vi "Write Registers to write.vi"(10 "Registers to write":T1[](array[typedef]), 11 "Device in":refnum<class "PIC-Device.lvclass">) -> (3 "Device out":refnum<class "PIC-Device.lvclass">)   [LabVIEW 2020, in "PIC-Device.lvclass"]
uses:
  PIC-Device.lvclass
  Controls/Register to Write.ctl
  PIC-Device.lvclass/PIC-Device.ctl
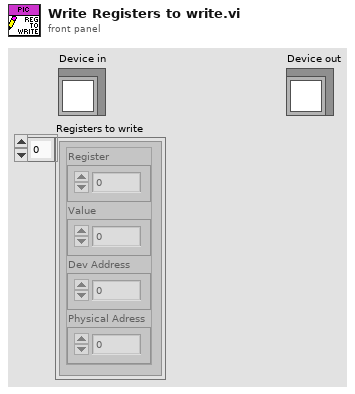
[diagram p1: front panel]
types:
  T1 = typedef "PIC-Device.lvclass/Register to Write.ctl" = cluster{"Register":u32, "Value":u32, "Dev Address":u32, "Physical Adress":u32}
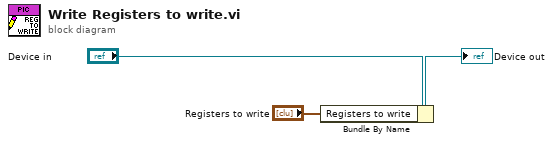
[diagram p0: block diagram]
diagram:
  n1 = Bundle By Name(cluster="Device in", "Registers to write"="Registers to write") -> (→"Device out":refnum<class "PIC-Device.lvclass">)
